vi "test A Future That Isnt Cancelled Shows Not Cancelled To Promise.vi"(8 "error in (no error)":errorcluster, 11 "TestCase in":refnum<class "Cancellation Tests.lvclass">) -> (0 "error out":errorcluster, 3 "TestCase out":refnum<class "Cancellation Tests.lvclass">)   [LabVIEW 2017]
uses:
  Cancellation Tests.lvclass
  <vilib>/addons/_JKI Toolkits/VI Tester/TestCase.llb/TestCase.lvclass
  Futures/Futures.lvlib
  Futures/Future/Future.lvclass
  Futures/Promise/Promise.lvclass
  C:/Program Files (x86)/National Instruments/LabVIEW 2017/vi.lib/addons/_JKI Toolkits/VI Tester/TestCase.llb/TestCase.lvclass
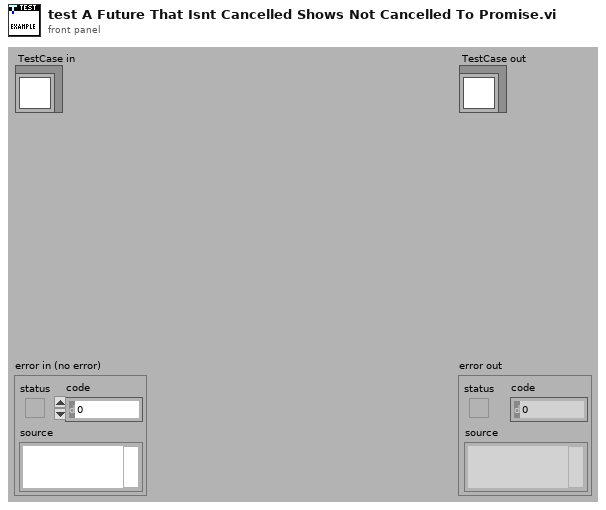
[diagram p1: front panel]
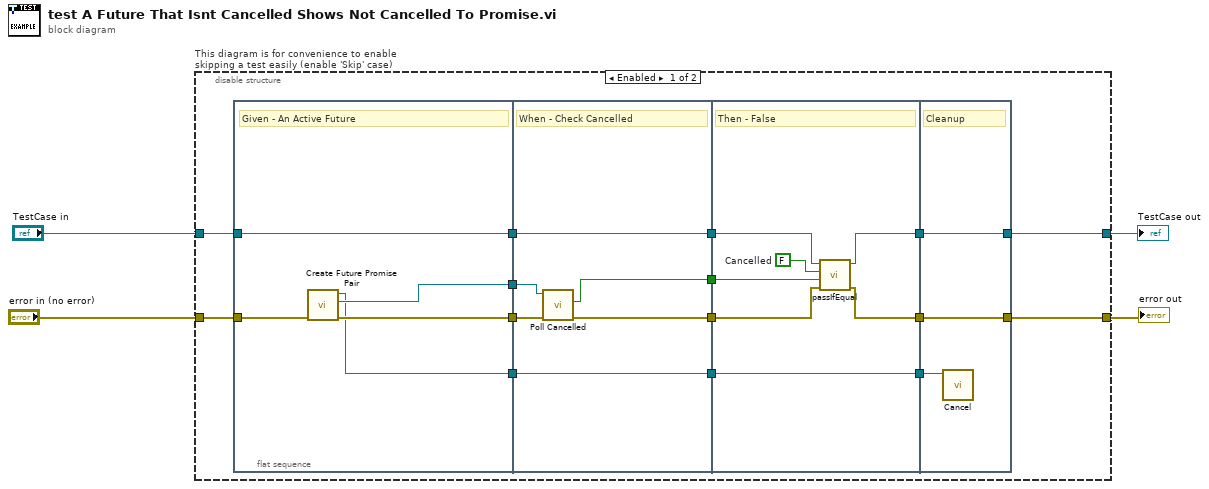
[diagram p0: block diagram]
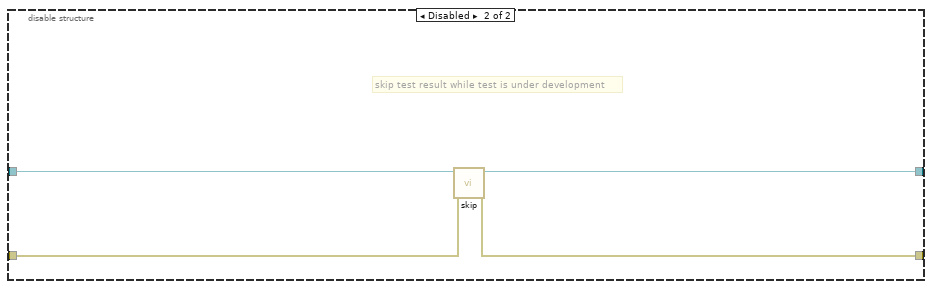
[diagram p2: hidden frame]
diagram:
  n1 = disable-structure "This diagram is for convenience to enable skipping a test easily (enable 'Skip' case)" shown="Enabled" {
    disable-tunnel: "TestCase in" -> [w14 w44]
    disable-tunnel: [w12 w42] -> w1
    disable-tunnel: [w11 w43] -> w3
    disable-tunnel: "error in (no error)" -> [w13 w41]
    frame Enabled {
      n2 = flat-sequence {
        tunnel: w13 -> [w23]
        tunnel: w14 -> [w24]
        tunnel: [w24] -> w19
        tunnel: [w22] -> w10
        tunnel: [w21] -> w9
        tunnel: [w20] -> w7
        tunnel: [w30] -> w18
        tunnel: [w27] -> w17
        tunnel: w19 -> [w30]
        tunnel: w10 -> [w29]
        tunnel: w9 -> [w28]
        tunnel: [w26] -> w8
        tunnel: w7 -> [w25]
        tunnel: [w25] -> w6
        tunnel: [w36] -> w16
        tunnel: [w34] -> w15
        tunnel: w18 -> [w37]
        tunnel: w17 -> [w35]
        tunnel: w8 -> [w33]
        tunnel: w6 -> [w31]
        tunnel: [w31] -> w5
        tunnel: [w39] -> w11
        tunnel: [w40] -> w12
        tunnel: w16 -> [w40]
        tunnel: w15 -> [w39]
        tunnel: w5 -> [w38]
        frame #0 {
          # "Given - An Active Future"
          n3 = call "Create Future Promise Pair.vi"("error in (no error)"=w23) -> ("error out"=w22:errorcluster, "Promise out"=w21:refnum<class "Promise.lvclass">, "Future out"=w20:refnum<class "Future.lvclass">)  [unwired: 8 in]
        }
        frame #1 {
          # "When - Check Cancelled"
          n4 = call "Poll Cancelled.vi"("error in (no error)"=w29, "Promise in"=w28) -> ("error out"=w27:errorcluster, "Cancelled"=w26:bool)  [unwired: 7 in, 1 out]
        }
        frame #2 {
          w32 = FALSE  # Cancelled
          # "Then - False"
          n5 = call-dynamic "passIfEqual.vi"("error in (no error)"=w35, "y"=w33, "x"=w32, "TestCase in"=w37) -> ("error out"=w34:errorcluster, "TestCase out"=w36:refnum<class "Cancellation Tests.lvclass">)  [unwired: 6 in]
        }
        frame #3 {
          # "Cleanup"
          n6 = call "Cancel.vi"("Future in"=w38) -> ()  [unwired: 10 in, 1 out]
        }
      }
    }
    frame Disabled {
      # "skip test result while test is under development"
      n7 = call <vilib>:"skip.vi"("error in (no error)"=w41, "TestCase in"=w44) -> ("error out"=w43:errorcluster, "TestCase out"=w42:refnum<class "Cancellation Tests.lvclass">)  [unwired: 8 in]
    }
  }
  "error out" <- w3
  "TestCase out" <- w1
